vi "LVIS_SendToBF.vi"(8 "Error In":errorcluster, 11 "Data":string) -> (0 "Error out":errorcluster)   [LabVIEW 2015]
doc: "Sends the event data to the backup file."
uses:
  Ctrls/LVIS_Msg State.ctl
  Globals/LVIS_IsGlobal.vi
  Globals/LVIS_DcGlobals.vi
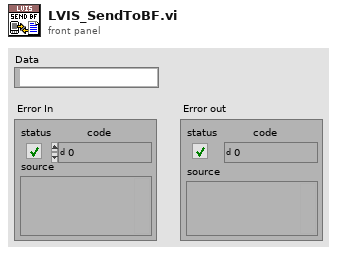
[diagram p1: front panel]
types:
  T1 = enum16{"open", "replace", "create", "open or create", "replace or create", "replace or create with confirmation"}
  T2 = typedef "LVIS_Msg State.ctl" = enum16{"None", "Offline", "Online", "Backup Full"}
  T3 = cluster{"DCIP":string, "BackupFile":string, "ErrorLog":string, "FilePosition":string}
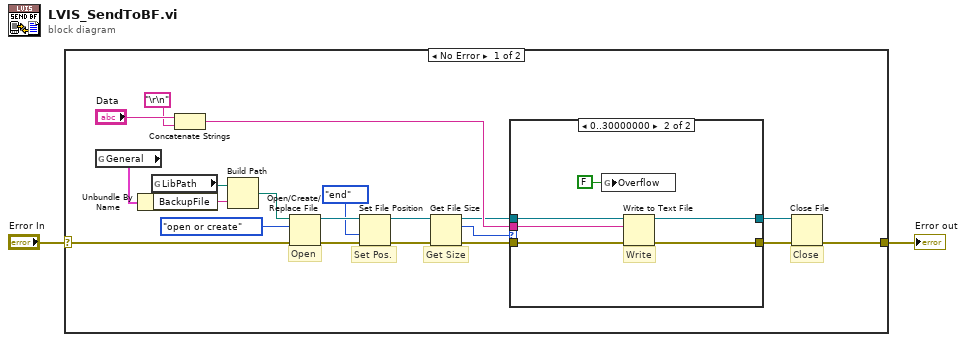
[diagram p0: block diagram]
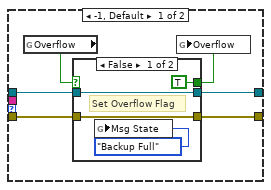
[diagram p2: hidden frame]
diagram:
  n1 = case shown="No Error" "Error In" {
    selector: "Error In" -> [w22 w42]
    tunnel: [w18 w42] -> w1
    frame No Error {
      # "Get Size"
      # "Set Pos."
      # "Close"
      # "Open"
      n2 = global read "LVIS_DcGlobals.vi" "General"() -> (w10:T3)
      n3 = Unbundle By Name(w10) -> ("BackupFile"=w11:string)
      n4 = global read "LVIS_IsGlobal.vi" "LibPath"() -> (w9:path)
      n5 = Concatenate Strings("Data", "\r\n") -> (w12:string)
      n6 = Build Path(base path=w9, name or relative path=w11) -> (appended path=w8:path)
      n7 = Open/Create/Replace File(file path (use dialog)=w8, error in=w22, operation (0:open)=T1."open or create") -> (refnum out=w16:refnum<file>, error out=w17:errorcluster)  [unwired: 3 in, 1 out]
      n8 = Set File Position(refnum=w16, from (0:start)=enum16{"start", "end", "current"}."end", error in=w17) -> (refnum out=w6:refnum<file>, error out=w7:errorcluster)  [unwired: 1 in]
      n9 = Get File Size(file=w6, error in=w7) -> (refnum out=w4:refnum<file>, size (in bytes)=w3:i64, 0:w5:errorcluster)
      n10 = case shown="0..30000000" w3 {
        tunnel: [w24 w38] -> w20
        tunnel: [w27 w37] -> w19
        tunnel: w12 -> [_ w40]
        tunnel: w5 -> [w25 w41]
        tunnel: w4 -> [w28 w39]
        frame -1, Default {
          n11 = global read "LVIS_DcGlobals.vi" "Overflow"() -> (w26:bool)
          n12 = case shown="False" w26 {
            selector: w26 -> [_ w33]
            tunnel: w28 -> [w32 w35]
            tunnel: [w32 w35] -> w27
            tunnel: w25 -> [w31 w34]
            tunnel: [w31 w34] -> w24
            tunnel: [TRUE w33] -> w23
            frame False {
              # "Set Overflow Flag"
              n13 = global write "LVIS_DcGlobals.vi" "Msg State"(LVIS_Msg_State."Backup Full" ("Msg State")) -> ()
            }
            frame True {
            }
          }
          n14 = global write "LVIS_DcGlobals.vi" "Overflow"(w23) -> ()
        }
        frame 0..30000000 {
          # "Write"
          n15 = global write "LVIS_DcGlobals.vi" "Overflow"(FALSE ("Overflow")) -> ()
          n16 = Write to Text File(file (use dialog)=w39, text=w40, error in=w41) -> (refnum out=w37:refnum<file>, error out=w38:errorcluster)  [unwired: 1 in, 1 out]
        }
      }
      n17 = Close File(refnum=w19, error in=w20) -> (error out=w18:errorcluster)  [unwired: 1 out]
    }
    frame Error {
    }
  }
  "Error out" <- w1
